vi "Controller Write Outputs.vi"(0 "PS Setpoint Variables":refnum<k21>[](array[refnum]), 1 "PS ON-OFF Variables":refnum<k21>[](array[refnum]), 3 "PS Setpoints":dbl[](array[numeric]), 4 "PS ON-OFF (per PS Rack)":u8[](array[numeric]), 5 "error in (no error)":errorcluster) -> (19 "error out":errorcluster)   [LabVIEW 2011, in "Controller VIs.lvlib"]
doc: "Writes all output variables to Actuation chassis."
uses:
  Controller VIs.lvlib
  Controller Write FXP20.5.vi
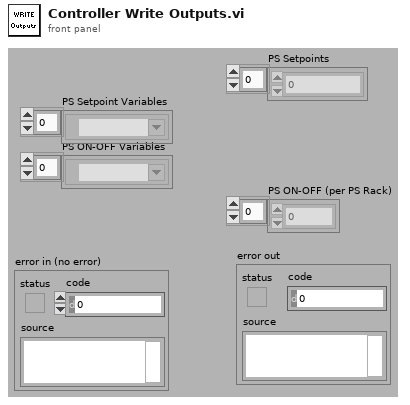
[diagram p1: front panel]
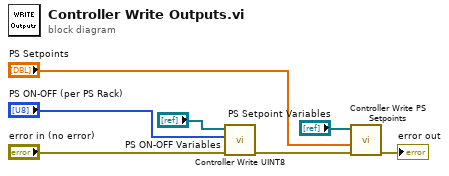
[diagram p0: block diagram]
diagram:
  n1 = call "Controller Write UINT8.vi"("error in (no error)"="error in (no error)", "Values"="PS ON-OFF (per PS Rack)", "Variables"="PS ON-OFF Variables") -> ("error out"=w3:errorcluster)  [unwired: 8 in]
  n2 = call "Controller Write PS Setpoints.vi"("PS Setpoint Variables"="PS Setpoint Variables", "PS Setpoints"="PS Setpoints", "error in (no error)"=w3) -> ("error out"=→"error out":errorcluster)  [unwired: 7 in]
